vi "saveData.vi"(8 "error in (no error)":errorcluster, 11 "reference in":refnum<class "Items Controller.lvclass">) -> (0 "error out":errorcluster, 3 "reference out":refnum<class "Items Controller.lvclass">)   [LabVIEW 2016, in "Items Controller.lvclass"]
uses:
  Items Controller.lvclass
  APP/excelFile_class/fileType.ctl
  APP/excelFile_class/excelFile.lvclass
  File Controller_llb/File Controller.lvclass
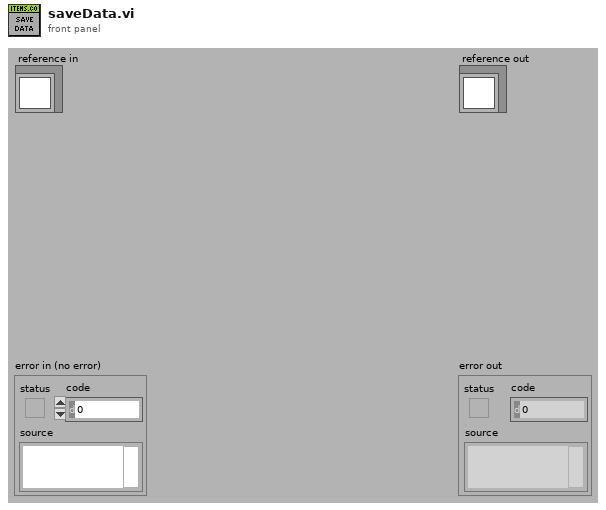
[diagram p1: front panel]
types:
  T1 = typedef "excelFile.lvclass/fileType.ctl" = enum16{"devices", "items", "partsTracking", "TSR"}
  T2 = typedef "Items Controller.lvclass/ObjectAttributesRef.ctl" = refnum<data-value>
  T3 = typedef "Items Controller.lvclass/ObjectAttributes.ctl" = cluster{"MyAttribute":dbl, "data":string[][][], "file_controller_ref":refnum<class "File Controller.lvclass">, "checkIN_ref":refnum<class "checkIN.lvclass">, "checkOUT_ref":refnum<class "checkOUT.lvclass">, "item_ref":refnum<class "item.lvclass">}
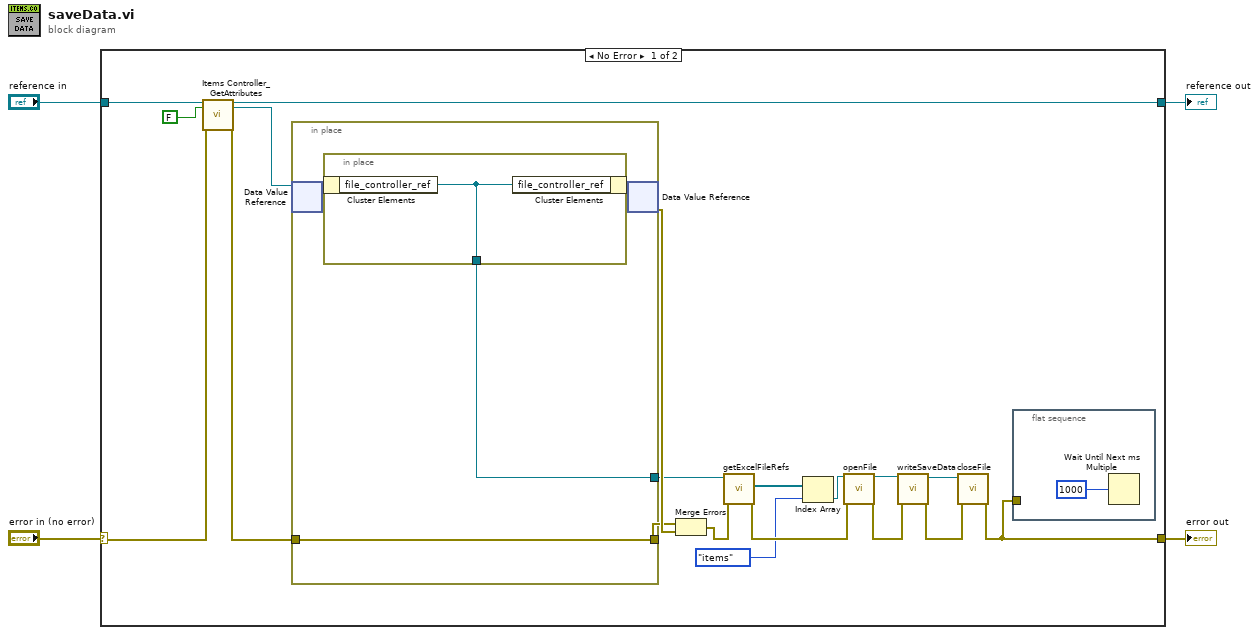
[diagram p0: block diagram]
diagram:
  n1 = case shown="No Error" "error in (no error)" {
    selector: "error in (no error)" -> [w19 w31]
    tunnel: [w5 w31] -> w3
    tunnel: [w17 w30] -> w1
    tunnel: "reference in" -> [w21 w30]
    frame No Error {
      n2 = call "Items Controller_GetAttributes.vi"("reference in"=w21, "return data? (T)"=FALSE, "error in (no error)"=w19) -> ("reference out"=w17:refnum<class "Items Controller.lvclass">, "attributes ref"=w16:T2, "error out"=w18:errorcluster)  [unwired: 13 in, 1 out]
      n3 = in-place {
        in-place-border: w18 -> [w26]
        in-place-border: [w26] -> w22
        in-place-border: [w25] -> w9
        n4 = in-place-dvr #1(w16) -> (w27:T3)  [unwired: 1 out]
        n5 = in-place {
          in-place-border: [w29] -> w25
          n6 = in-place-cluster #2(w27) -> ("file_controller_ref"=w29:refnum<class "File Controller.lvclass">)
          n7 = in-place-cluster #2("file_controller_ref"=w29) -> (w28:T3)
        }
        n8 = in-place-dvr #1(w28) -> (w23:errorcluster)  [unwired: 1 out]
      }
      n9 = Merge Errors(w22, w23) -> (w11:errorcluster)
      n10 = call "getExcelFileRefs.vi"("error in (no error)"=w11, "reference in"=w9) -> ("error out"=w10:errorcluster, "excelFile_refs"=w8:refnum<class "excelFile.lvclass">[])  [unwired: 7 in, 1 out]
      n11 = Index Array(array=w8, index=fileType."items" ("fileType")) -> (element=w7:refnum<class "excelFile.lvclass">)
      n12 = call "openFile.vi"("reference in"=w7, "error in (no error)"=w10) -> ("reference out"=w15:refnum<class "excelFile.lvclass">, "error out"=w13:errorcluster)  [unwired: 16 in]
      n13 = call "writeSaveData.vi"("error in (no error)"=w13, "reference in"=w15) -> ("error out"=w12:errorcluster, "reference out"=w14:refnum<class "excelFile.lvclass">)  [unwired: 8 in]
      n14 = call "closeFile.vi"("error in (no error)"=w12, "reference in"=w14) -> ("error out"=w5:errorcluster)  [unwired: 8 in, 1 out]
      n15 = flat-sequence {
        tunnel: w5 -> [_]
        frame #0 {
          n16 = Wait Until Next ms Multiple(millisecond multiple=u32 1000) -> ()  [unwired: 1 out]
        }
      }
    }
    frame Error {
    }
  }
  "error out" <- w3
  "reference out" <- w1
